vi "QmixTC_Test.vi"() -> ()   [LabVIEW 2010]
uses:
  labbCAN_Bus_API/labbCAN_Bus_API.lvlib
  labbCAN_Controller_API/labbCAN_Controller_API.lvlib
panel:
  out "Signalverlaufsdiagramm":dbl(graph)
  out "Actual Value":dbl
  in  "Stopp":bool
  out "error out":errorcluster caption="Fehler (Ausgang)"
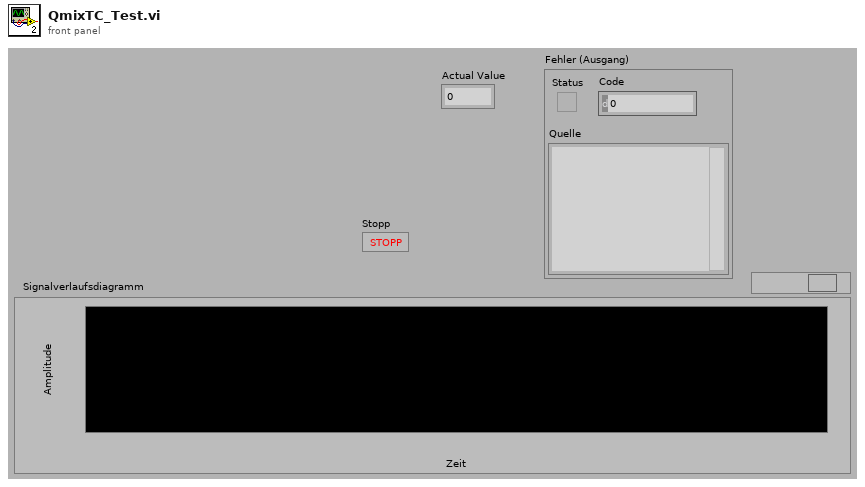
[diagram p1: front panel]
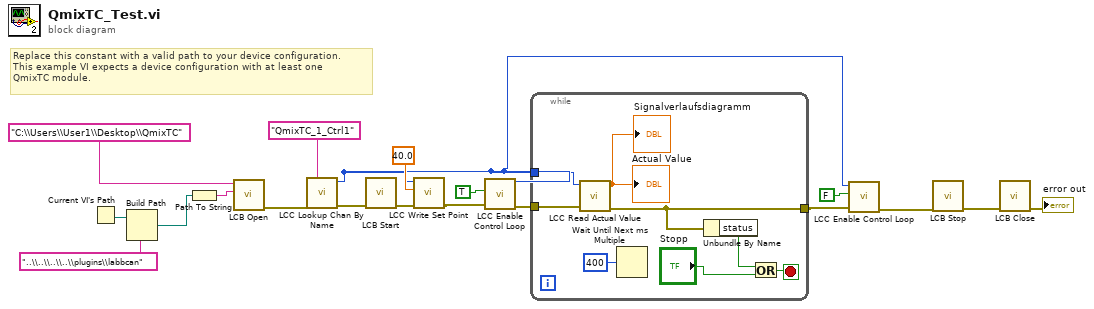
[diagram p0: block diagram]
diagram:
  # "Replace this constant with a valid path to your device configuration.\nThis example VI expects a device configuration with at least one\nQmixTC module."
  n1 = Current VI's Path() -> (path=w8:path)
  n2 = Build Path(base path=w8, name or relative path="..\\..\\..\\..\\plugins\\labbcan" ("Name oder relativer Pfad")) -> (appended path=w17:path)
  n3 = Path To String(path=w17) -> (string=w15:string)
  n4 = call "LCB Open.vi"("PluginSearchPath"=w15, "Device Configuration Path"="C:\\Users\\User1\\Desktop\\QmixTC" ("Name oder relativer Pfad")) -> ("error out"=w7:errorcluster)  [unwired: 9 in]
  n5 = call "LCC Lookup Chan By Name.vi"("error in (no error)"=w7, "Channel Name"="QmixTC_1_Ctrl1") -> ("error out"=w13:errorcluster, "Channel Handle"=w4:i64)  [unwired: 8 in]
  n6 = call "LCB Start.vi"("error in (no error)"=w13) -> ("error out"=w12:errorcluster)  [unwired: 10 in]
  n7 = call "LCC Write Set Point.vi"("error in (no error)"=w12, "Setpoint"=40.0, "Channel Handle"=w4) -> ("error out"=w1:errorcluster)  [unwired: 8 in]
  n8 = call "LCC Enable Control Loop.vi"("error in (no error)"=w1, "Enable"=TRUE, "ChanHdl"=w4) -> ("error out"=w9:errorcluster)  [unwired: 8 in]
  n9 = while {
    tunnel: w9 -> [w26]
    tunnel: [w25] -> w2
    tunnel: w4 -> [w21]
    stop <- w22 stop-if-true
    n10 = call "LCC Read Actual Value.vi"("error in (no error)"=w26, "Channel Handle"=w21) -> ("error out"=w25:errorcluster, "Actual Value"=→"Actual Value" →"Signalverlaufsdiagramm":dbl)  [unwired: 8 in]
    n11 = Wait Until Next ms Multiple(millisecond multiple=u32 400 ("Vielfache von ms")) -> ()  [unwired: 1 out]
    n12 = Unbundle By Name(w25) -> ("status"=w24:bool)
    n13 = Or(x=w24, y="Stopp") -> (x .or. y?=w22:bool)
  }
  n14 = call "LCC Enable Control Loop.vi"("error in (no error)"=w2, "Enable"=FALSE, "ChanHdl"=w4) -> ("error out"=w5:errorcluster)  [unwired: 8 in]
  n15 = call "LCB Stop.vi"("error in (no error)"=w5) -> ("error out"=w18:errorcluster)  [unwired: 10 in]
  n16 = call "LCB Close.vi"("error in (no error)"=w18) -> ("error out"=→"error out":errorcluster)  [unwired: 10 in]
